vi "enumerateStaticDependencies.vi"(8 "error in (no error)":errorcluster, 11 "Instrument":refnum<class "Instrument.lvclass">) -> (0 "error out":errorcluster, 2 "Static Dependencies":refnum<class "Dependency.lvclass">[](array[class]), 3 "Instrument out":refnum<class "Instrument.lvclass">)   [LabVIEW 2019, in "Instrument.lvclass"]
doc: "JKI State Machine Objects (SMO) 1.3.0.56\nJKI - JKI\nCopyright (c) 2017, JKI"
uses:
  Instrument.lvclass
  C:/Program Files (x86)/National Instruments/LabVIEW 2019/vi.lib/JKI/JKI SMO/SMO/SMO.lvclass
  <vilib>/JKI/JKI SMO/Dependency/Dependency.lvclass
  Logger.Error/Logger.Error.lvclass
  C:/Users/patrick/Documents/GitHub/Instrument-Framework/lvsrc/SMOs/Logger/Logger.lvclass
  Logger.PGSQL/Logger.PGSQL.lvclass
  Logger.Error/Logger.Error.lvclass/Logger.Error.ctl
  <userlib>/LevyLab/RemoteControl/RemoteControl.lvclass
  <vilib>/JKI/JKI SMO/SMO/SMO.lvclass
  Logger/Logger.lvclass
panel:
  # "For instructions on how to use the JKI State Machine Objects, examples and video tutorials, visit:\nhttp://jki.net/state-machine-objects/\n\nJKI State Machine Objects™\nhttp://jki.net/state-machine-objects/\nCopyright (C) 2005-2015, JKI <info@jki.net>\nALL RIGHTS RESERVED"
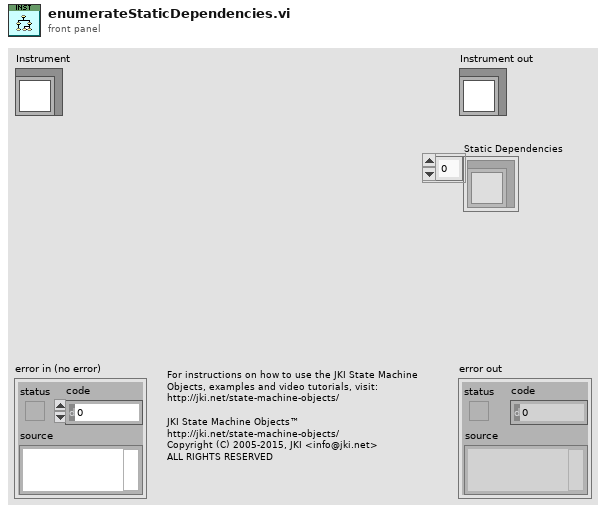
[diagram p1: front panel]
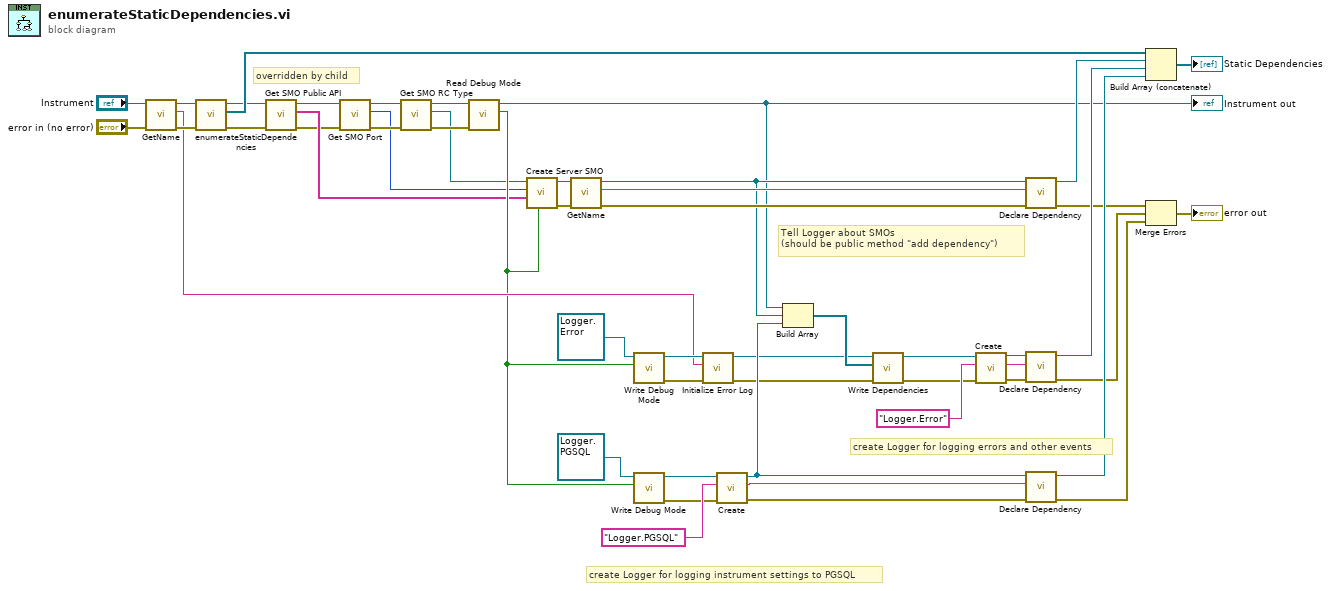
[diagram p0: block diagram]
diagram:
  # "Tell Logger about SMOs\n(should be public method \"add dependency\")"
  # "create Logger for logging errors and other events"
  # "create Logger for logging instrument settings to PGSQL"
  # "overridden by child"
  n1 = call <vilib>:"GetName.vi"("error in (no error)"="error in (no error)", "SMO"="Instrument") -> ("error out"=w47:errorcluster, "Name"=w12:string, "SMO out"=w48:refnum<class "Instrument.lvclass">)  [unwired: 6 in, 1 out]
  n2 = call-parent "enumerateStaticDependencies.vi"("error in (no error)"=w47, "SMO"=w48) -> ("error out"=w7:errorcluster, "Static Dependencies"=w22:refnum<class "Dependency.lvclass">[], "SMO out"=w8:refnum<class "Instrument.lvclass">)  [unwired: 7 in]
  n3 = call-dynamic "Get SMO Public API.vi"("error in (no error)"=w7, "Instrument in"=w8) -> ("error out"=w9:errorcluster, "Commands"=w10:string[], "Instrument out"=w35:refnum<class "Instrument.lvclass">)  [unwired: 7 in]
  n4 = call-dynamic "Get SMO Port.vi"("error in (no error)"=w9, "Instrument in"=w35) -> ("error out"=w5:errorcluster, "Port"=w2:u16, "Instrument out"=w6:refnum<class "Instrument.lvclass">)  [unwired: 7 in]
  n5 = call-dynamic "Get SMO RC Type.vi"("error in (no error)"=w5, "Instrument in"=w6) -> ("error out"=w4:errorcluster, "Dependencies.RemoteControl"=w1:refnum<class "RemoteControl.lvclass">, "Instrument out"=w3:refnum<class "Instrument.lvclass">)  [unwired: 7 in]
  n6 = call-dynamic "Read Debug Mode.vi"("error in (no error)"=w4, "Instrument in"=w3) -> ("Debug Mode?"=w11:bool, "Instrument out"=w20:refnum<class "Instrument.lvclass">)  [unwired: 7 in, 1 out]
  "Instrument out" <- w20
  n7 = call <userlib>:"Create Server SMO.vi"("Debug Mode?"=w11, "Commands"=w10, "Port"=w2, "RemoteControl in"=w1) -> ("error out"=w24:errorcluster, "RemoteControl out"=w25:refnum<class "RemoteControl.lvclass">)  [unwired: 6 in]
  n8 = call <vilib>:"GetName.vi"("error in (no error)"=w24, "SMO"=w25) -> ("error out"=w27:errorcluster, "Name"=w28:string, "SMO out"=w21:refnum<class "RemoteControl.lvclass">)  [unwired: 6 in, 1 out]
  n9 = call "Write Debug Mode.vi"("Debug Mode?"=w11, "Logger in"=refnum<class "Logger.Error.lvclass"> refnum ("Logger.Error.lvclass")) -> ("error out"=w16:errorcluster, "Logger out"=w15:refnum<class "Logger.Error.lvclass">)  [unwired: 8 in]
  n10 = call "Write Debug Mode.vi"("Debug Mode?"=w11, "Logger in"=refnum<class "Logger.PGSQL.lvclass"> refnum ("Logger.PGSQL.lvclass")) -> ("error out"=w38:errorcluster, "Logger out"=w37:refnum<class "Logger.PGSQL.lvclass">)  [unwired: 8 in]
  n11 = call "Initialize Error Log.vi"("error in (no error)"=w16, "Application Name"=w12, "Logger.Error in"=w15) -> ("error out"=w13:errorcluster, "Logger.Error out"=w14:refnum<class "Logger.Error.lvclass">)  [unwired: 7 in]
  n12 = call <vilib>:"Create.vi"("error in (no error)"=w38, "Subsystem Name (optional)"="Logger.PGSQL" ("Name"), "SMO"=w37) -> ("error out"=w40:errorcluster, "SMO name"=w17:string, "SMO out"=w30:refnum<class "Logger.PGSQL.lvclass">)  [unwired: 6 in]
  n13 = Build Array(w20, w21, w30) -> (w29:refnum<class "SMO.lvclass">[])
  n14 = call "Write Dependencies.vi"("error in (no error)"=w13, "SMOs"=w29, "Logger.Error in"=w14) -> ("error out"=w31:errorcluster, "Logger.Error out"=w32:refnum<class "Logger.Error.lvclass">)  [unwired: 7 in]
  n15 = call <vilib>:"Create.vi"("error in (no error)"=w31, "Subsystem Name (optional)"="Logger.Error" ("Name"), "SMO"=w32) -> ("error out"=w42:errorcluster, "SMO name"=w18:string, "SMO out"=w43:refnum<class "Logger.Error.lvclass">)  [unwired: 6 in]
  n16 = call <vilib>:"Declare Dependency.vi"("error in (no error)"=w27, "Name"=w28, "Type"=w21) -> ("error out"=w26:errorcluster, "Dependency out"=w33:refnum<class "Dependency.lvclass">)  [unwired: 7 in]
  n17 = call <vilib>:"Declare Dependency.vi"("error in (no error)"=w42, "Name"=w18, "Type"=w43) -> ("error out"=w23:errorcluster, "Dependency out"=w45:refnum<class "Dependency.lvclass">)  [unwired: 7 in]
  n18 = call <vilib>:"Declare Dependency.vi"("error in (no error)"=w40, "Name"=w17, "Type"=w30) -> ("error out"=w34:errorcluster, "Dependency out"=w36:refnum<class "Dependency.lvclass">)  [unwired: 7 in]
  n19 = Build Array (concatenate)(w22, w33, w45, w36) -> (→"Static Dependencies":refnum<class "Dependency.lvclass">[])
  n20 = Merge Errors(w26, w23, w34) -> (→"error out":errorcluster)
